vi "p01 - Creating Sub VI.vi"() -> ()   [LabVIEW 2025]
panel:
  out "Result":dbl
  in  "Operation":enum16{"Add", "Sub", "Mult", "Div"}(ring)
  in  "B":dbl
  in  "A":dbl
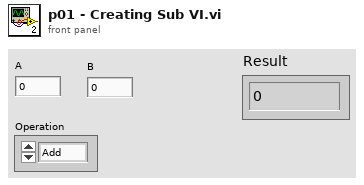
[diagram p1: front panel]
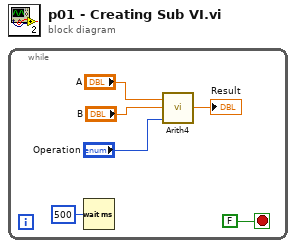
[diagram p0: block diagram]
diagram:
  n1 = while {
    stop <- FALSE stop-if-true
    n2 = Wait (ms)(milliseconds to wait=u32 500) -> ()  [unwired: 1 out]
    n3 = call "Arith4.vi"("Operation"="Operation", "B"="B", "A"="A") -> ("Output"=→"Result":dbl)  [unwired: 8 in]
  }
